vi "TCPread8bytes.vi"(8 "Error in":errorcluster, 10 "timeout ms (25000)":i32, 11 "connection ID in":refnum<k5>) -> (0 "Error out":errorcluster, 2 "string out":string, 3 "connection ID out":refnum<k5>)   [LabVIEW 2013]
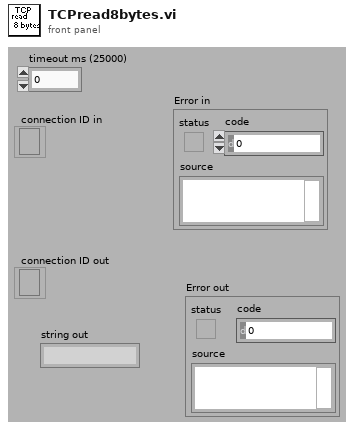
[diagram p1: front panel]
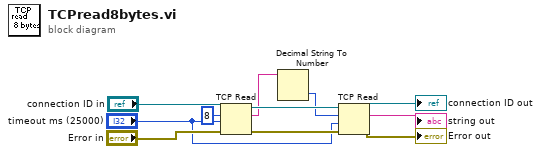
[diagram p0: block diagram]
diagram:
  n1 = TCP Read ("TCP Read Command")(connection ID="connection ID in", bytes to read=8, error in (no error)="Error in", 9:"timeout ms (25000)") -> (connection ID out=w10:refnum<k5>, data out=w3:string, error out=w11:errorcluster)  [unwired: 1 out]
  n2 = Decimal String To Number(string=w3) -> (number=w9:i32)  [unwired: 3 out]
  n3 = TCP Read(connection ID=w10, bytes to read=w9, error in (no error)=w11, 9:"timeout ms (25000)") -> (connection ID out=→"connection ID out":refnum<k5>, data out=→"string out":string, error out=→"Error out":errorcluster)  [unwired: 1 out]
